vi "ERIO RT Process State Variables.vi"(6 "Supervisory Variables In":T4={"Alarm Threshold"=0.0, "Shutdown"=FALSE, "Enable SNS Alarm"=FALSE, "Enable SNS Stage Notification"=FALSE, "Enable SQS Notification"=FALSE, "Enable S3 TDMS Signal Capture"=FALSE, "Enable SystemLink Signal Capture"=FALSE, "Capture Signal"=FALSE, "Server Update"=FALSE, "AWS Access Key"="AKIAINLDO2Y2PDFEWDOQ", "AWS Secret Key"="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", "Phone Number"="+15037066913", "Region"=enum."us-west-2", "AWS SQS Queue"="mynicloud-demotest2", "AWS S3 Bucket"="mynicloud-demotest2"}, 7 "RT State In":T1, 8 "error in (no error)":errorcluster, 9 "AWS Variables In":T6, 11 "EEISysLink.lvclass In":refnum<class "EEISysLink.lvclass">) -> (0 "error out":errorcluster, 1 "AWS Variables Out":T6, 3 "EEISysLink.lvclass Out":refnum<class "EEISysLink.lvclass">, 4 "Supervisory Variables Out":T4={"Alarm Threshold"=0.0, "Shutdown"=FALSE, "Enable SNS Alarm"=FALSE, "Enable SNS Stage Notification"=FALSE, "Enable SQS Notification"=FALSE, "Enable S3 TDMS Signal Capture"=FALSE, "Enable SystemLink Signal Capture"=FALSE, "Capture Signal"=FALSE, "Server Update"=FALSE, "AWS Access Key"="AKIAINLDO2Y2PDFEWDOQ", "AWS Secret Key"="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", "Phone Number"="+15037066913", "Region"=enum."us-west-2", "AWS SQS Queue"="mynicloud-demotest2", "AWS S3 Bucket"="mynicloud-demotest2"}, 5 "RT State Out":T1)   [LabVIEW 2017]
doc: "Process conveyor simulation state variables. Update input values from the process, process them as needed for this control iteration, and update the SystemLink server worker tags. \n\nJames Tillett P.E.\nEndeavor Engineering Inc.\nwww.endeavoreng.com"
uses:
  Class EEISysLink/EEISysLink.lvclass
  Controls/ERIO AWS Toolkit Variables.ctl
  <vilib>/AWS Toolkit/SQS/Queue/Queue.lvclass
  <vilib>/AWS Toolkit/SNS/Phone Number/Phone Number.lvclass
  <vilib>/AWS Toolkit/S3/Bucket/Bucket.lvclass
  Controls/ERIO Supervisory Variables.ctl
  <vilib>/AWS Toolkit/Core/HTTP Request/Region.ctl
  Controls/ERIO RT State Variables.ctl
  Controls/ERIO SystemStates.ctl
  Controls/ERIO Queue Data.ctl
  Controls/ERIO Worker Variables.ctl
  Class EEISysLink/Controls/SL Tag Scope.ctl
  <vilib>/Utility/error.llb/Error Cluster From Error Code.vi
  <vilib>/rvi/errors/niLvFpgaAdjustHostInterfaceError.vi
  <vilib>/measure/mascope.llb/Amplitude and Levels 1 chan.vi
  <vilib>/rvi/interface/nirviReadWriteControl/nirviReadWriteControl.xnode
  <vilib>/rvi/interface/nirviMethod/nirviMethod.xnode
  <vilib>/measure/NI_MAPro.lvlib
  <vilib>/rvi/interface/Simulation/niFpgaSimulationCallBeginRW.vi
  <vilib>/FPGAPlugInAG/Dynamic/niLvFpga_ReadFifo_Dynamic.vi
  <vilib>/rvi/errors/niLvFpgaMergeErrorWithErrorCode.vi
  NiFpgaLv.dll
  <vilib>/AWS Toolkit/Core/HTTP Request/HTTP Request.lvclass
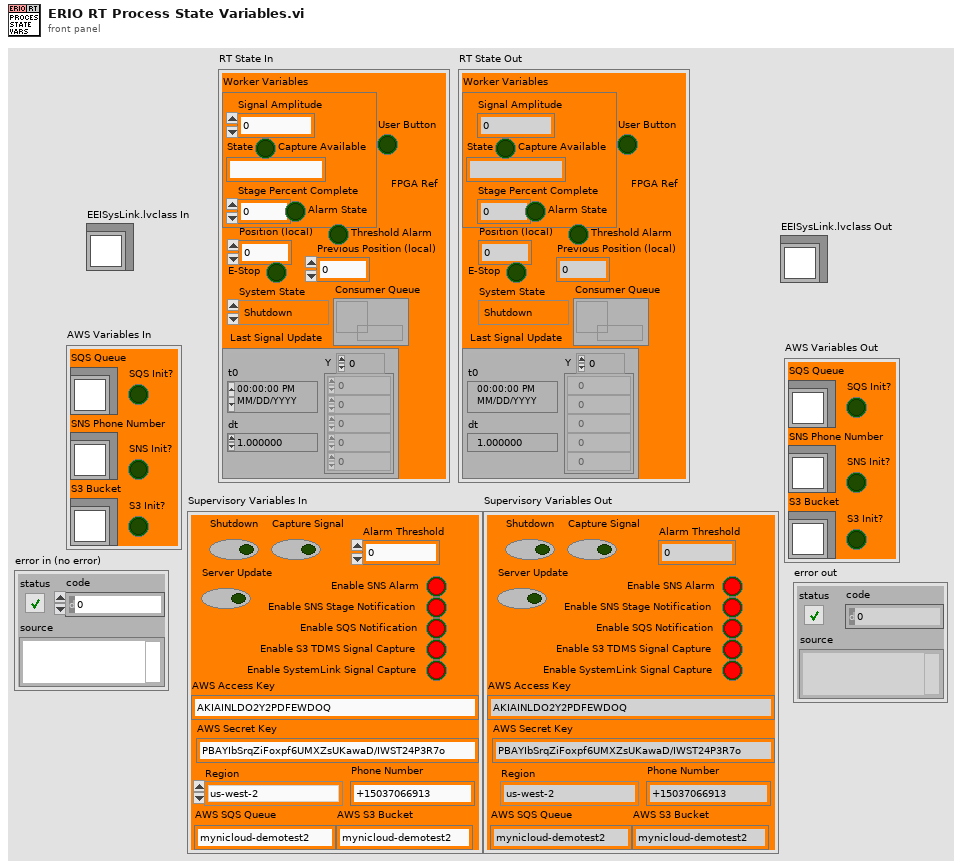
[diagram p1: front panel]
types:
  T1 = typedef "ERIO RT State Variables.ctl" = cluster{"Position (local)":i16, "E-Stop":bool, "System State":T2, "FPGA Ref":refnum<k20>, "Previous Position (local)":i16, "Consumer Queue":refnum<queue>, "Worker Variables":T3, "Threshold Alarm":bool, "User Button":bool, "Last Signal Update":waveform(dbl)}
  T2 = typedef "ERIO SystemStates.ctl" = enum16{"Shutdown", "E-STOP", "Reset Process", "Stage 1", "Stage 2", "Stage 3", "Alarm State"}
  T3 = typedef "ERIO Worker Variables.ctl" = cluster{"Signal Amplitude":dbl, "State":string, "Stage Percent Complete":dbl, "Alarm State":bool, "Capture Available":bool}
  T4 = typedef "ERIO Supervisory Variables.ctl" = cluster{"Alarm Threshold":dbl, "Shutdown":bool, "Enable SNS Alarm":bool, "Enable SNS Stage Notification":bool, "Enable SQS Notification":bool, "Enable S3 TDMS Signal Capture":bool, "Enable SystemLink Signal Capture":bool, "Capture Signal":bool, "Server Update":bool, "AWS Access Key":string, "AWS Secret Key":string, "Phone Number":string, "Region":T5, "AWS SQS Queue":string, "AWS S3 Bucket":string}
  T5 = typedef "NI_AWS_Core.lvlib/HTTP Request.lvclass/Region.ctl" = enum16{"us-east-1", "us-east-2", "us-west-1", "us-west-2", "ap-northeast-1", "ap-northeast-2", "ap-southeast-1", "ap-southeast-2", "ca-central-1", "eu-central-1", "eu-west-1", "eu-west-2", "sa-east-1"}
  T6 = typedef "ERIO AWS Toolkit Variables.ctl" = cluster{"SQS Queue":refnum<class "Queue.lvclass">, "SNS Phone Number":refnum<class "Phone Number.lvclass">, "S3 Bucket":refnum<class "Bucket.lvclass">, "SQS Init?":bool, "S3 Init?":bool, "SNS Init?":bool}
  T7 = typedef "EEISysLink.lvclass/SL Tag Scope.ctl" = enum16{"Local", "Server"}
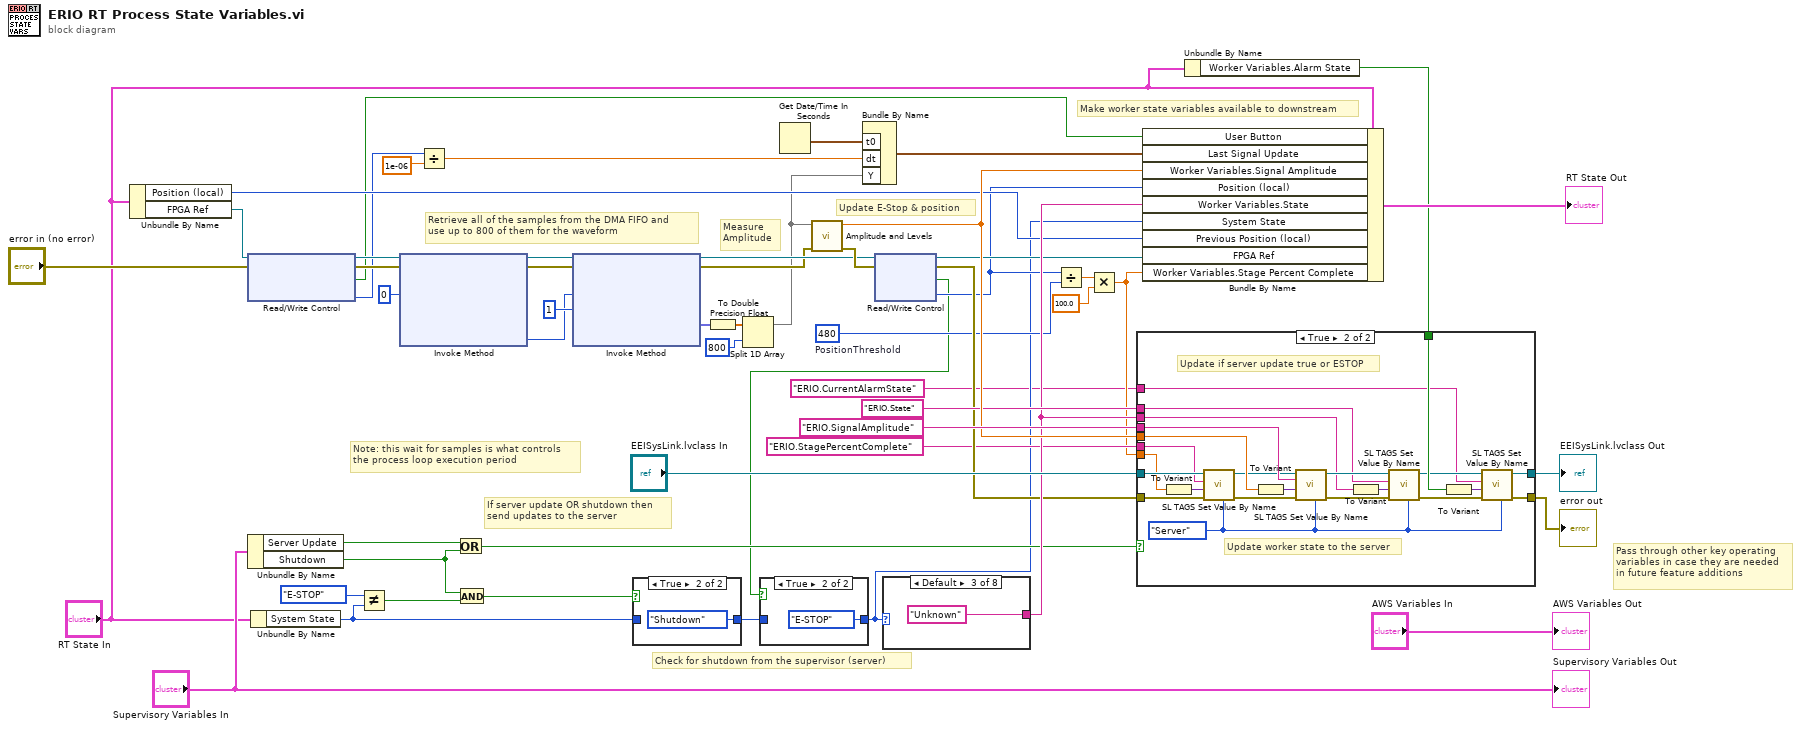
[diagram p0: block diagram]
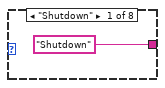
[diagram p5: hidden frame]
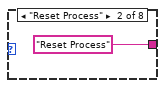
[diagram p6: hidden frame]
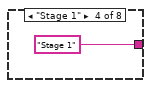
[diagram p7: hidden frame]
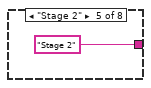
[diagram p8: hidden frame]
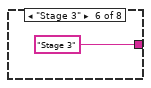
[diagram p9: hidden frame]
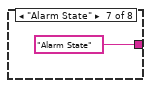
[diagram p10: hidden frame]
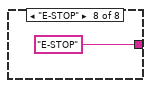
[diagram p11: hidden frame]
diagram:
  w36 = i16 480  # PositionThreshold
  # "Note: this wait for samples is what controls\nthe process loop execution period"
  # "If server update OR shutdown then\nsend updates to the server"
  # "Check for shutdown from the supervisor (server)"
  # "Make worker state variables available to downstream"
  # "Pass through other key operating\nvariables in case they are needed\nin future feature additions"
  # "Update E-Stop & position"
  # "Measure\nAmplitude"
  # "Retrieve all of the samples from the DMA FIFO and \nuse up to 800 of them for the waveform"
  n1 = Unbundle By Name("RT State In") -> ("Position (local)"=w39:i16, "FPGA Ref"=w8:refnum<k20>)
  n2 = xnode "Read/Write Control"("FPGA VI Reference In"=w8, "error in"="error in (no error)") -> ("FPGA VI Reference Out"=w19:refnum<k20>, "error out"=w18:errorcluster, "User Notification"=w7:bool, "Signal dt (uSec)"=w3:u32)
  n3 = Unbundle By Name("Supervisory Variables In") -> ("Server Update"=w42:bool, "Shutdown"=w22:bool)
  n4 = Unbundle By Name("RT State In") -> ("System State"=w24:T2)
  n5 = Not Equal?(x=ERIO_SystemStates."E-STOP" ("System State"), y=w24) -> (x != y?=w23:bool)
  n6 = xnode "Invoke Method"("FPGA VI Reference In"=w19, "error in"=w18, "Number of Elements"=u32 0) -> ("FPGA VI Reference Out"=w17:refnum<k20>, "error out"=w16:errorcluster, "Elements Remaining"=w20:u32)  [unwired: 1 in, 1 out]
  n7 = Divide(x=w3, y=1e-06) -> (x/y=w2:dbl)
  n8 = Or(x=w42, y=w22) -> (x .or. y?=w41:bool)
  n9 = And(x=w22, y=w23) -> (x .and. y?=w21:bool)
  n10 = xnode "Invoke Method"("FPGA VI Reference In"=w17, "error in"=w16, "Number of Elements"=w20, "Timeout (ms)"=1) -> ("FPGA VI Reference Out"=w38:refnum<k20>, "error out"=w37:errorcluster, "Data"=w29:fxp<+/-,24,5>[])  [unwired: 1 out]
  n11 = case shown="True" w21 {
    tunnel: w24 -> [w55 _]
    tunnel: [w55 ERIO_SystemStates."Shutdown" ("System State")] -> w27
    frame False {
    }
    frame True {
    }
  }
  n12 = To Double Precision Float(number=w29) -> (double precision float=w45:dbl[])
  n13 = Split 1D Array(array=w45, index=800) -> (first subarray=w6:dbl[])  [unwired: 1 out]
  n14 = Get Date/Time In Seconds() -> (seconds since 1Jan1904=w5:timestamp)
  n15 = call-poly <vilib>:"Amplitude and Levels.vi"("error in (no error)"=w37, "signal in"=w6) -> ("error out"=w52:errorcluster, "amplitude"=w51:dbl)  [unwired: 6 in, 2 out]
  n16 = Bundle By Name("t0"=w5, "dt"=w2, "Y"=w6) -> (w1:waveform(dbl))  [unwired: 1 in]
  n17 = xnode ("Read/Write Control")("FPGA VI Reference In"=w38, "error in"=w52) -> ("FPGA VI Reference Out"=w40:refnum<k20>, "error out"=w43:errorcluster, "E-Stop"=w26:bool, "Position"=w35:i16)
  n18 = case shown="True" w26 {
    tunnel: w27 -> [w57 _]
    tunnel: [w57 ERIO_SystemStates."E-STOP" ("System State")] -> w28
    frame False {
    }
    frame True {
    }
  }
  n19 = case shown="Default" w28 {
    tunnel: ["Shutdown" "Reset Process" "Unknown" "Stage 1" "Stage 2" "Stage 3" "Alarm State" "E-STOP"] -> w44
    frame "Shutdown" {
    }
    frame "Reset Process" {
    }
    frame Default {
    }
    frame "Stage 1" {
    }
    frame "Stage 2" {
    }
    frame "Stage 3" {
    }
    frame "Alarm State" {
    }
    frame "E-STOP" {
    }
  }
  n20 = Divide(x=w35, y=w36) -> (x/y=w34:dbl)
  n21 = Multiply(x=w34, y=100.0) -> (x*y=w31:dbl)
  n22 = Bundle By Name(cluster="RT State In", "User Button"=w7, "Last Signal Update"=w1, "Worker Variables.Signal Amplitude"=w51, "Position (local)"=w35, "Worker Variables.State"=w44, "System State"=w28, "Previous Position (local)"=w39, "FPGA Ref"=w40, "Worker Variables.Stage Percent Complete"=w31) -> (→"RT State Out":T1)
  n23 = Unbundle By Name("RT State In") -> ("Worker Variables.Alarm State"=w10:bool)
  n24 = case shown="True" w41 {
    tunnel: "EEISysLink.lvclass In" -> [w68 w82]
    tunnel: "ERIO.SignalAmplitude" -> [_ w90]
    tunnel: w51 -> [_ w89]
    tunnel: "ERIO.State" -> [_ w85]
    tunnel: [w67 w71] -> w49
    tunnel: [w68 w72] -> w47
    tunnel: w44 -> [_ w84]
    tunnel: w43 -> [w67 w81]
    tunnel: "ERIO.StagePercentComplete" -> [_ w80]
    tunnel: w31 -> [_ w79]
    tunnel: w10 -> [_ w75]
    tunnel: "ERIO.CurrentAlarmState" -> [_ w69]
    frame False {
      # "Server update not requested"
    }
    frame True {
      w70 = SL_Tag_Scope."Server" ("Tag Scope")
      # "Update if server update true or ESTOP"
      # "Update worker state to the server"
      n25 = To Variant(anything=w79) -> (Variant=w83:variant)
      n26 = call-dynamic "SL TAGS Set Value By Name.vi"("Tag Scope"=w70, "error in (no error)"=w81, "Value"=w83, "Tag Name"=w80, "EEISysLink in"=w82) -> ("error out"=w77:errorcluster, "EEISysLink out"=w78:refnum<class "EEISysLink.lvclass">)  [unwired: 5 in]
      n27 = To Variant(anything=w89) -> (Variant=w91:variant)
      n28 = call-dynamic "SL TAGS Set Value By Name.vi"("Tag Scope"=w70, "error in (no error)"=w77, "Value"=w91, "Tag Name"=w90, "EEISysLink in"=w78) -> ("error out"=w87:errorcluster, "EEISysLink out"=w88:refnum<class "EEISysLink.lvclass">)  [unwired: 5 in]
      n29 = To Variant(anything=w84) -> (Variant=w86:variant)
      n30 = call-dynamic "SL TAGS Set Value By Name.vi"("Tag Scope"=w70, "error in (no error)"=w87, "Value"=w86, "Tag Name"=w85, "EEISysLink in"=w88) -> ("error out"=w73:errorcluster, "EEISysLink out"=w74:refnum<class "EEISysLink.lvclass">)  [unwired: 5 in]
      n31 = To Variant(anything=w75) -> (Variant=w76:variant)
      n32 = call-dynamic "SL TAGS Set Value By Name.vi"("Tag Scope"=w70, "error in (no error)"=w73, "Value"=w76, "Tag Name"=w69, "EEISysLink in"=w74) -> ("error out"=w71:errorcluster, "EEISysLink out"=w72:refnum<class "EEISysLink.lvclass">)  [unwired: 5 in]
    }
  }
  "EEISysLink.lvclass Out" <- w47
  "error out" <- w49
  "AWS Variables Out" <- "AWS Variables In"
  "Supervisory Variables Out" <- "Supervisory Variables In"
